vi "1A-z-invdist.vi"(8 "err in":errorcluster, 9 "F(z)":dbl) -> (0 "err out":errorcluster caption="err  out", 1 "F(z)":dbl, 2 "z":dbl)   [LabVIEW 2010, in "lv_02.lvlib"]
uses:
  <vilib>/gmath/statdist.llb/Normal Inverse CDF.vi
  lv_02.lvlib
  <vilib>/gmath/NI_Gmath.lvlib
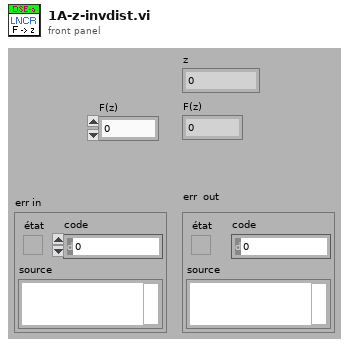
[diagram p1: front panel]
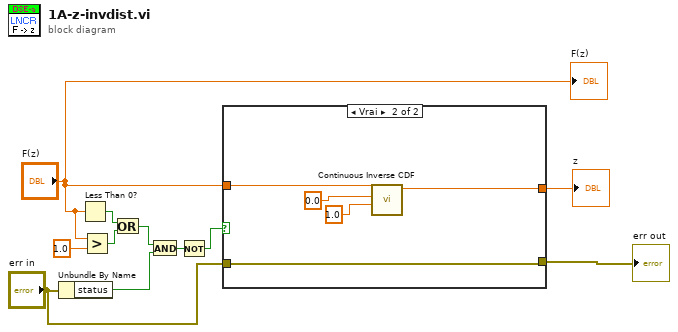
[diagram p0: block diagram]
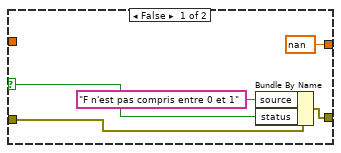
[diagram p2: hidden frame]
diagram:
  n1 = Unbundle By Name("err in") -> ("status"=w5:bool)
  n2 = Less Than 0?(x="F(z)") -> (x < 0?=w7:bool)
  n3 = Greater?(x="F(z)", y=1.0) -> (0:w8:bool)
  n4 = Or(x=w7, y=w8) -> (x .or. y?=w6:bool)
  n5 = And(x=w6, y=w5) -> (x .and. y?=w4:bool)
  n6 = Not(x=w4) -> (.not. x?=w3:bool)
  n7 = case shown="Vrai" w3 {
    selector: w3 -> [w13 _]
    tunnel: "F(z)" -> [_ w19]
    tunnel: [nan ("x") w18] -> w11
    tunnel: "err in" -> [w14 w17]
    tunnel: [w15 w17] -> w1
    frame False {
      n8 = Bundle By Name(cluster=w14, "source"="F n'est pas compris entre 0 et 1", "status"=w13) -> (w15:errorcluster)
    }
    frame True {
      n9 = call-poly <vilib>:"Continuous Inverse CDF.vi"("std"=1.0 ("mean"), "mean"=0.0 ("x"), "cdf(x)"=w19) -> ("x"=w18:dbl)  [unwired: 7 in, 1 out]
    }
  }
  "z" <- w11
  "err out" <- w1
  "F(z)" <- "F(z)"
